vi "_Get Interfaces.vi"(8 "error in (no error)":errorcluster, 11 "Interfaceable in":refnum<class "Interfaceable.lvclass">) -> (0 "error out":errorcluster, 2 "Concrete Interfaces":refnum<class "IUnknown.lvclass">[](array[class]), 3 "Interfaceable out":refnum<class "Interfaceable.lvclass">)   [LabVIEW 2009, in "Interfaceable.lvclass"]
doc: "Returns an array of all the concrete interfaces implemented for the given interfaceable object. Classes that inherit from Interfacable must override this vi."
uses:
  Interfaceable.lvclass
  IUnknown Class/IUnknown.lvclass
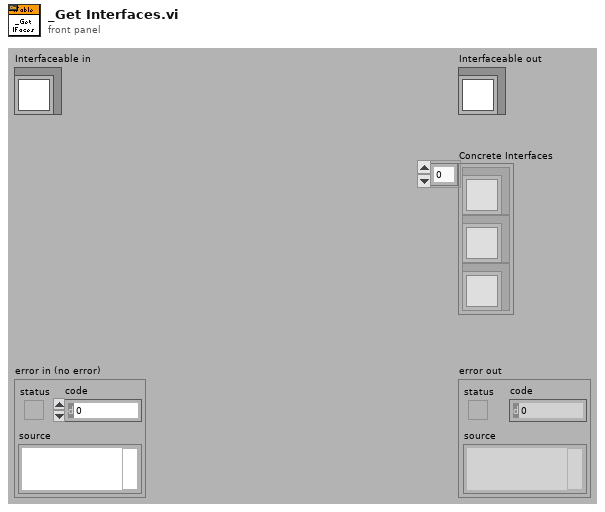
[diagram p1: front panel]
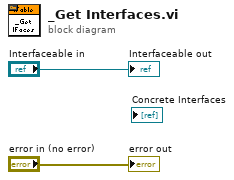
[diagram p0: block diagram]
diagram:
  "error out" <- "error in (no error)"
  "Interfaceable out" <- "Interfaceable in"
